vi "Response AutoControlRefHandler DataTypes.vi"() -> (3 "Unit Test Framework Results":T1)   [LabVIEW 2023]
uses:
  <vilib>/utf/common/utf_test_result_troll.ctl
  <vilib>/utf/common/utf_test_result.ctl
  <vilib>/utf/common/utf_test_result_failure.ctl
  <vilib>/utf/common/utf_test_comparison_operators.ctl
  <vilib>/utf/common/utf_vi_tag.ctl
  API Message/API Message.lvclass
  <vilib>/Utility/error.llb/DialogType.ctl
  <vilib>/httpClient/POSTBuffer.vi
  <vilib>/utf/NI_UnitTestFramework.lvlib
  Server/Server.lvclass
  <vilib>/httpClient/LabVIEWHTTPClient.lvlib
  <vilib>/Utility/Data Type/NI_Data Type.lvlib
panel:
  in  "Path Array":path[](array[path])=[path "C:/Program Files/National Instruments/CompactRIO", path "C:/Program Files/National Instruments/LabVIEW 2020", path "C:/Program Files/National Instruments/LabVIEW 2021", path "C:/Program Files/National Instruments/LabVIEW 2022", path "C:/Program Files/National Instruments/LabVIEW 2023", path "C:/Program Files/National Instruments/LabVIEW 2024", path "C:/Program Files/National Instruments/MAX", path "C:/Program Files/National Instruments/MXI", path "C:/Program Files/National Instruments/NI Controller Driver", path "C:/Program Files/National Instruments/NI Hardware Configuration", path "C:/Program Files/National Instruments/NI Package Manager", path "C:/Program Files/National Instruments/NI-DAQ", path "C:/Program Files/National Instruments/NI-PCNet", path "C:/Program Files/National Instruments/NI-QPXI", path "C:/Program Files/National Instruments/NI-Sync", path "C:/Program Files/National Instruments/NI-SyncBus", path "C:/Program Files/National Instruments/NI-SyncEnet", path "C:/Program Files/National Instruments/NI-TSU", path "C:/Program Files/National Instruments/PXI Platform Services", path "C:/Program Files/National Instruments/Real-Time Trace Viewer 2023", path "C:/Program Files/National Instruments/Shared"]
  in  "String Array":string[](array[string])=["C", "Program Files", "National Instruments"]
  in  "Boolean Array":bool[](array[boolean])=[FALSE, FALSE, FALSE, TRUE, FALSE, FALSE, TRUE, TRUE]
  in  "EXT Array":ext[](array[numeric])=[0.0, 3.456, 6.912, 10.368, 13.824, 17.279999999999999999, 20.736, 24.192, 27.648, 31.103999999999999999]
  in  "DBL Array":dbl[](array[numeric])=[0.0, 2.345, 4.69, 7.035, 9.38, 11.725000000000001, 14.07, 16.415000000000003, 18.76, 21.105]
  in  "SGL Array":sgl[](array[numeric])=[0.0, 1.234, 2.468, 3.702, 4.936, 6.17, 7.404, 8.638, 9.872, 11.106]
  in  "U64 Array":u64[](array[numeric])=[200000, 200001, 200002, 200003, 200004, 200005, 200006, 200007, 200008, 200009]
  in  "U32 Array":u32[](array[numeric])=[20000, 20001, 20002, 20003, 20004, 20005, 20006, 20007, 20008, 20009]
  in  "U16 Array":u16[](array[numeric])=[2000, 2001, 2002, 2003, 2004, 2005, 2006, 2007, 2008, 2009]
  in  "U8 Array":u8[](array[numeric])=[200, 201, 202, 203, 204, 205, 206, 207, 208, 209]
  in  "I64 Array":i64[](array[numeric])=[100000, 100001, 100002, 100003, 100004, 100005, 100006, 100007, 100008, 100009]
  in  "I32 Array":i32[](array[numeric])=[10000, 10001, 10002, 10003, 10004, 10005, 10006, 10007, 10008, 10009]
  in  "I16 Array":i16[](array[numeric])=[1000, 1001, 1002, 1003, 1004, 1005, 1006, 1007, 1008, 1009]
  in  "I8 Array":i8[](array[numeric])=[100, 101, 102, 103, 104, 105, 106, 107, 108, 109]
  in  "Path":path=path "C:/Program Files/National Instruments/LabVIEW 2020"
  in  "String":string="Hello, World!"
  in  "Boolean":bool
  in  "EXT":ext=11.0
  in  "DBL":dbl=10.0
  in  "SGL":sgl=9.0
  in  "U64":u8=8
  in  "I64":i8=4
  in  "U32":u8=7
  in  "I32":i8=3
  in  "U16":u8=6
  in  "I16":i8=2
  in  "U8":u8=5
  in  "I8":i8=1
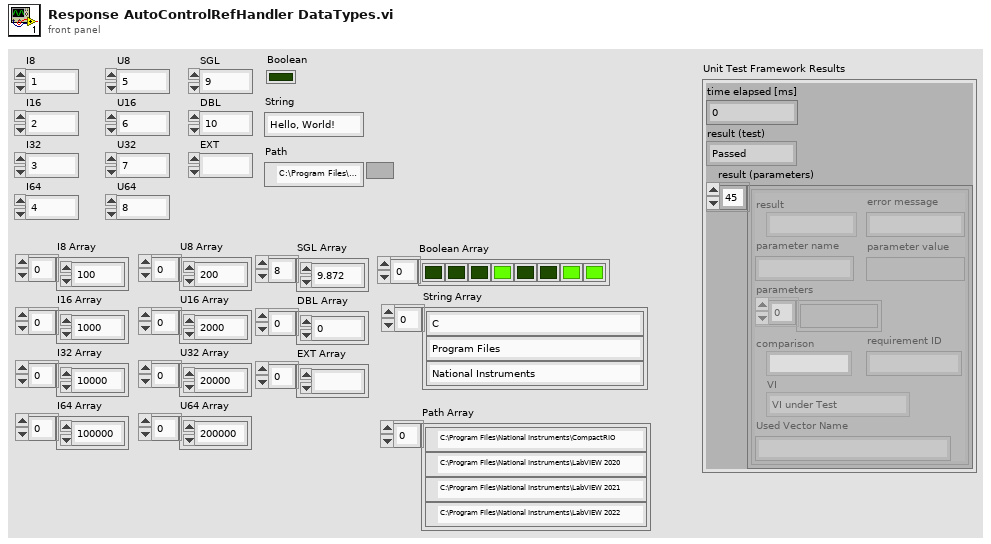
[diagram p1: front panel]
types:
  T1 = typedef "NI_UnitTestFramework.lvlib/utf_test_result_troll.ctl" = cluster{"time elapsed [ms]":u32, "result (test)":T2, "result (parameters)":T3[]}
  T2 = typedef "NI_UnitTestFramework.lvlib/utf_test_result.ctl" = enum16{"Passed", "Failed", "Error", "Skipped", "Not Processed"}
  T3 = typedef "NI_UnitTestFramework.lvlib/utf_test_result_failure.ctl" = cluster{"result":T2, "error message":string, "parameter name":string, "parameter value":variant, "parameters":variant[], "comparison":T4, "requirement ID":string, "VI":T5, "Used Vector Name":string}
  T4 = typedef "NI_UnitTestFramework.lvlib/utf_test_comparison_operators.ctl" = enum16{"=", "!=", ">", ">=", "<", "<=", "range", "symmetric tolerance", "asymmetric tolerance", "string contains", "string not contain", "array size", "string length", "array range", "by element", "array range (limit array)", "user-defined", "array contains", "array not contain", "vector length", "= (elm)", "!= (elm)", "= (case insensitive)", "!= (case insensitive)"}
  T5 = typedef "NI_UnitTestFramework.lvlib/utf_vi_tag.ctl" = enum16{"Setup VI", "VI under Test", "Teardown VI"}
  T6 = typedef "LabVIEWHTTPClient.lvlib/ClientHandle.ctl" = refnum<k1>
  T7 = typedef "DialogType.ctl" = u16
  T8 = typedef "NI_Data Type.lvlib/Data Type.ctl" = enum8{"Invalid Type", "Void", "I8", "I16", "I32", "I64", "U8", "U16", "U32", "U64", "Single Float", "Double Float", "Extended Float", "Single Complex", "Double Complex", "Extended Complex", "Enum U8", "Enum U16", "Enum U32", "Enum U64", "Single Float With Unit", "Double Float With Unit", "Extended Float With Unit", "Single Complex with Unit", "Double Complex with Unit", "Extended Complex with Unit", "Boolean", "String", "Path", "Picture", "Tag", "Array", "Cluster", "Variant", "LV Variant", "Waveform", "Timestamp", "Digital Waveform", "Digital Data", "ExpressData", "Refnum", "External Data", "VI", "Poly VI", "LabVIEW Class Instance", "Fixed Point", "Set Collection", "Map Collection"}
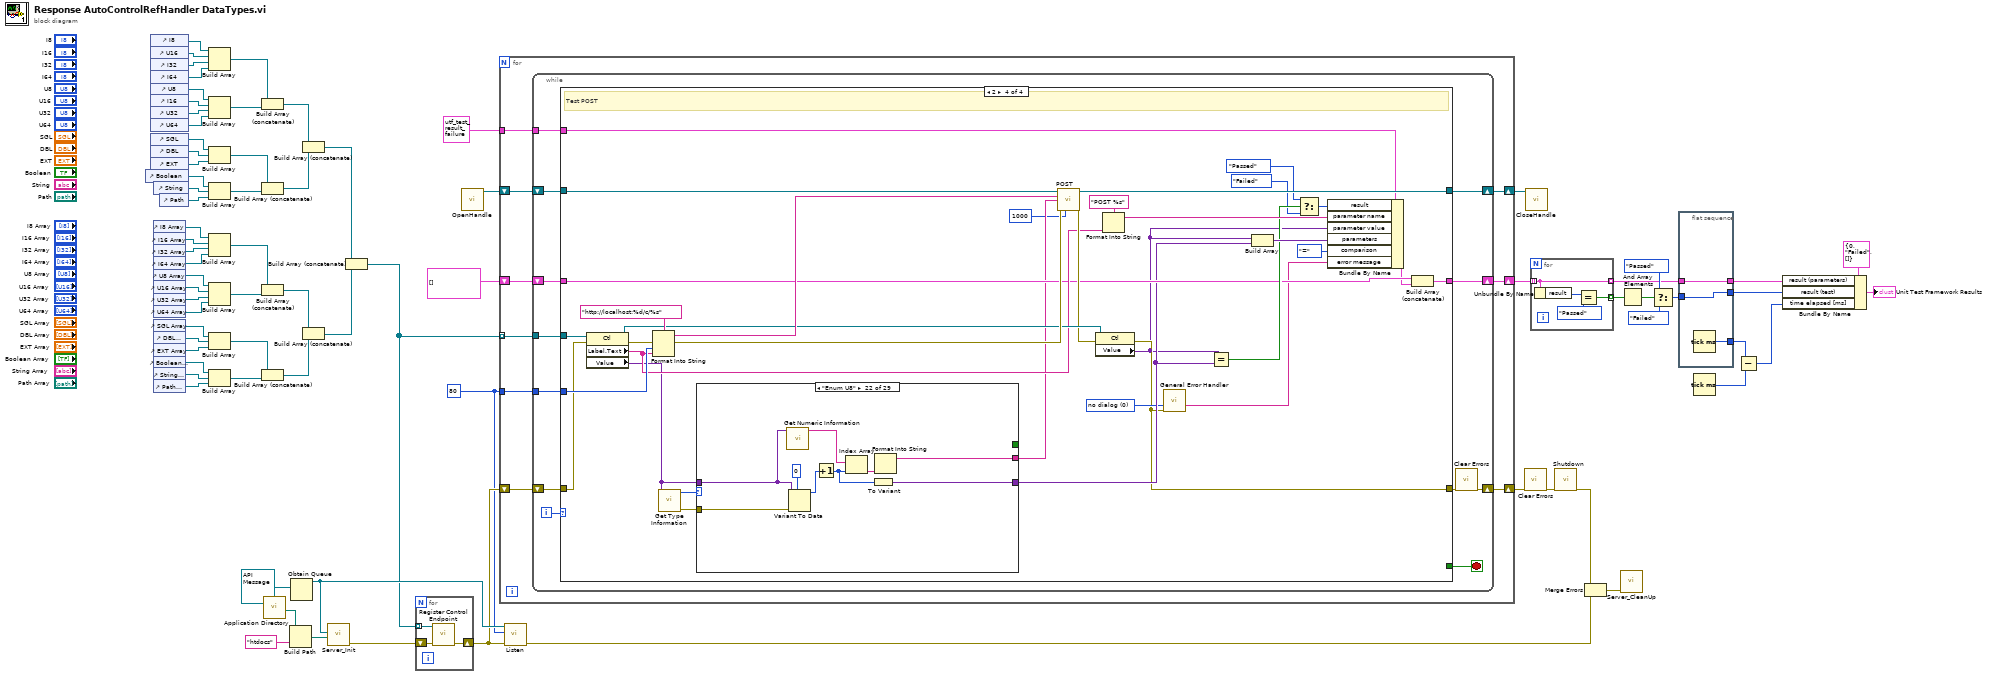
[diagram p0: block diagram]
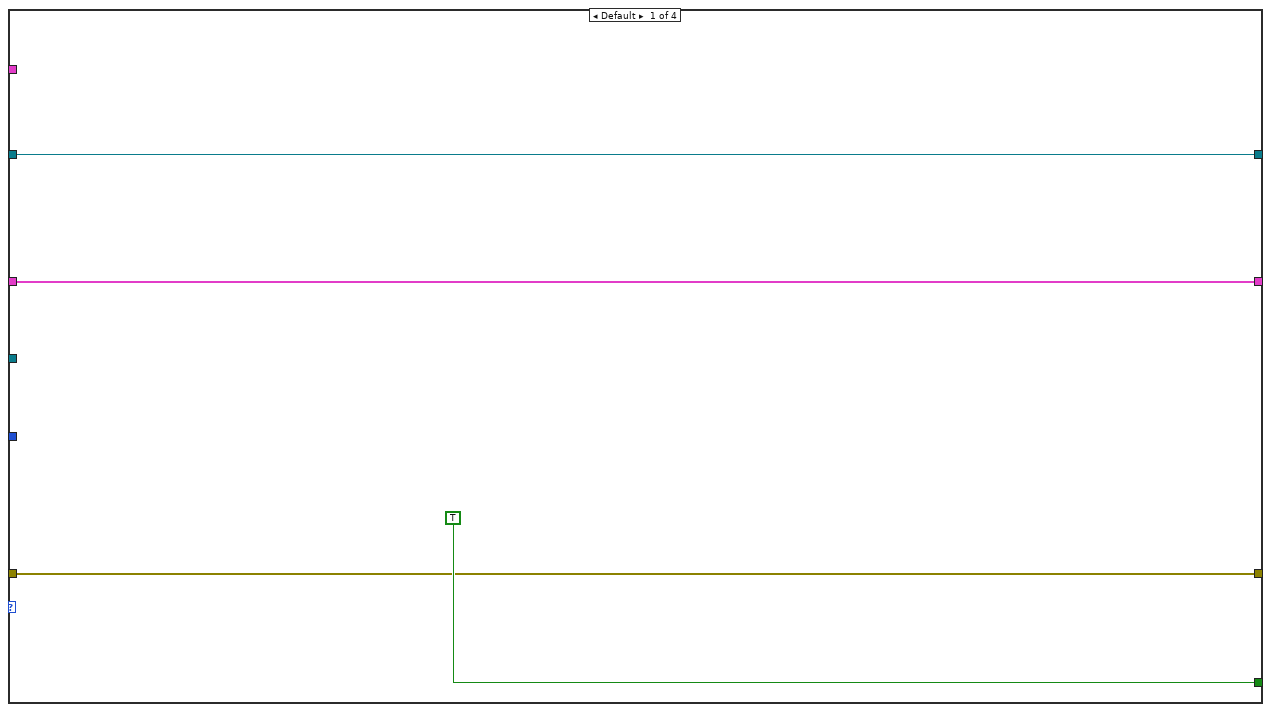
[diagram p2: hidden frame]
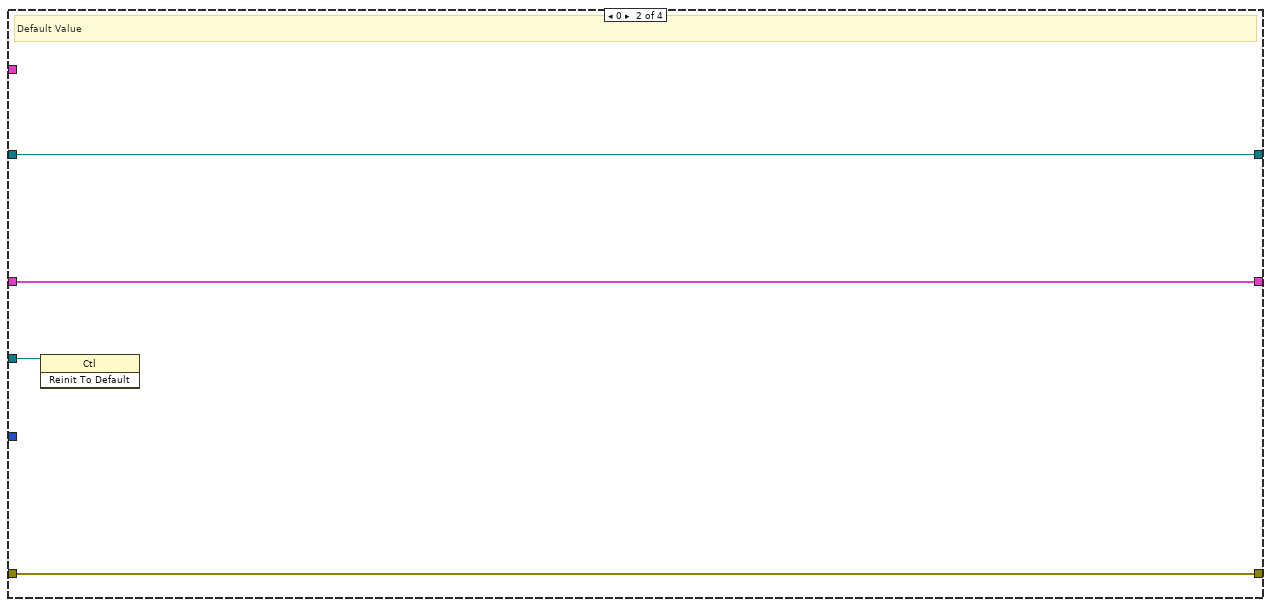
[diagram p3: hidden frame]
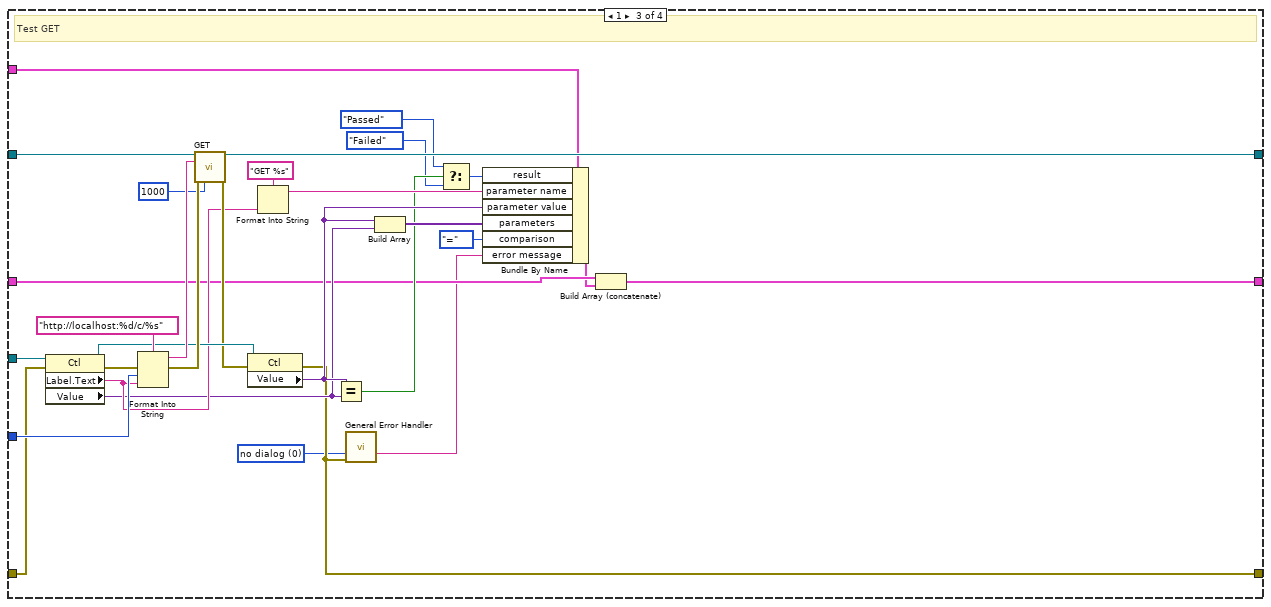
[diagram p4: hidden frame]
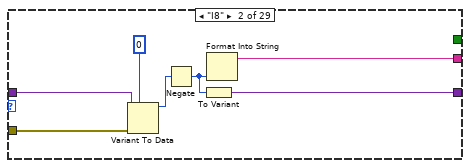
[diagram p6: hidden frame]
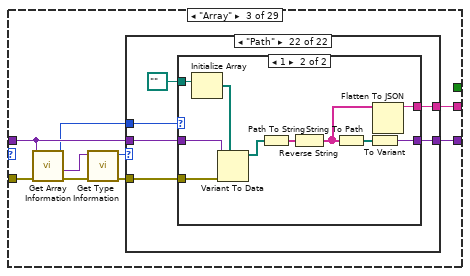
[diagram p7: hidden frame]
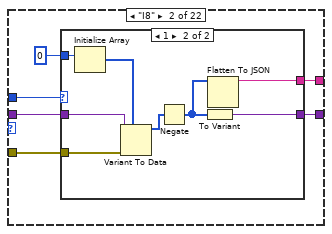
[diagram p9: hidden frame]
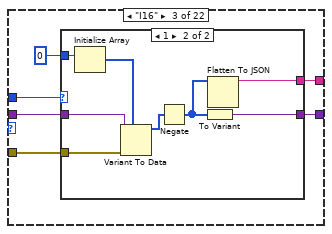
[diagram p11: hidden frame]
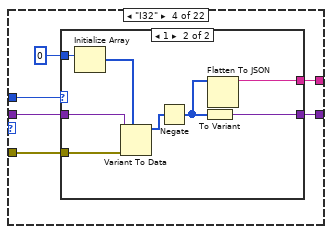
[diagram p13: hidden frame]
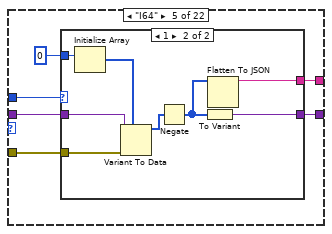
[diagram p15: hidden frame]
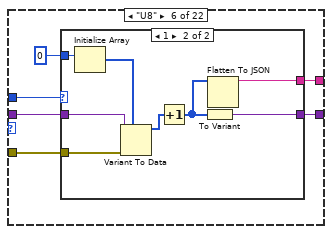
[diagram p17: hidden frame]
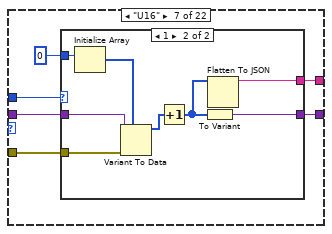
[diagram p19: hidden frame]
diagram:
  w33 = u16 80 ("Listen Port (80)")
  n1 = control-ref of="Boolean"() -> (w30:refnum<vi>)
  n2 = control-ref of="I8"() -> (w50:refnum<vi>)
  n3 = control-ref of="U16"() -> (w52:refnum<vi>)
  n4 = control-ref of="I32"() -> (w51:refnum<vi>)
  n5 = control-ref of="I64"() -> (w49:refnum<vi>)
  n6 = control-ref of="U8"() -> (w48:refnum<vi>)
  n7 = control-ref of="I16"() -> (w45:refnum<vi>)
  n8 = control-ref of="U32"() -> (w46:refnum<vi>)
  n9 = control-ref of="U64"() -> (w47:refnum<vi>)
  n10 = control-ref of="SGL"() -> (w35:refnum<vi>)
  n11 = control-ref of="DBL"() -> (w37:refnum<vi>)
  n12 = control-ref of="EXT"() -> (w36:refnum<vi>)
  n13 = control-ref of="String"() -> (w28:refnum<vi>)
  n14 = control-ref of="I8 Array"() -> (w8:refnum<vi>)
  n15 = control-ref of="I16 Array"() -> (w6:refnum<vi>)
  n16 = control-ref of="I32 Array"() -> (w7:refnum<vi>)
  n17 = control-ref of="I64 Array"() -> (w9:refnum<vi>)
  n18 = control-ref of="U8 Array"() -> (w10:refnum<vi>)
  n19 = control-ref of="U16 Array"() -> (w13:refnum<vi>)
  n20 = control-ref of="U32 Array"() -> (w12:refnum<vi>)
  n21 = control-ref of="U64 Array"() -> (w11:refnum<vi>)
  n22 = control-ref of="SGL Array"() -> (w16:refnum<vi>)
  n23 = control-ref of="DBL Array"() -> (w14:refnum<vi>)
  n24 = control-ref of="EXT Array"() -> (w15:refnum<vi>)
  n25 = control-ref of="Boolean Array"() -> (w17:refnum<vi>)
  n26 = control-ref of="String Array"() -> (w19:refnum<vi>)
  n27 = control-ref of="Path Array"() -> (w18:refnum<vi>)
  n28 = control-ref of="Path"() -> (w29:refnum<vi>)
  n29 = Build Array(w50, w52, w51, w49) -> (w67:refnum<vi>[])
  n30 = Build Array(w48, w45, w46, w47) -> (w66:refnum<vi>[])
  n31 = Build Array(w35, w37, w36) -> (w26:refnum<vi>[])
  n32 = Build Array(w30, w28, w29) -> (w27:refnum<vi>[])
  n33 = Build Array(w8, w6, w7, w9) -> (w4:refnum<vi>[])
  n34 = Build Array(w10, w13, w12, w11) -> (w5:refnum<vi>[])
  n35 = Build Array(w16, w14, w15) -> (w21:refnum<vi>[])
  n36 = Build Array(w17, w19, w18) -> (w20:refnum<vi>[])
  n37 = Build Array (concatenate)(w67, w66) -> (w24:refnum<vi>[])
  n38 = Build Array (concatenate)(w26, w27) -> (w25:refnum<vi>[])
  n39 = Build Array (concatenate)(w4, w5) -> (w23:refnum<vi>[])
  n40 = Build Array (concatenate)(w21, w20) -> (w22:refnum<vi>[])
  n41 = call <vilib>:"Application Directory.vi"() -> ("Application Directory"=w71:path)
  n42 = Build Path(base path=w71, name or relative path="htdocs" ("section")) -> (appended path=w70:path)
  n43 = Obtain Queue(element data type=refnum<class "API Message.lvclass"> refnum ("API Message.lvclass")) -> (queue out=w64:refnum<queue>)  [unwired: 4 in, 2 out]
  n44 = Build Array (concatenate)(w24, w25) -> (w2:refnum<vi>[])
  n45 = Build Array (concatenate)(w23, w22) -> (w3:refnum<vi>[])
  n46 = call "Server_Init.vi"("Static Data Folder"=w70, "API Queue"=w64) -> ("error out"=w68:errorcluster)  [unwired: 8 in, 1 out]
  n47 = Build Array (concatenate)(w2, w3) -> (w1:refnum<vi>[])
  n48 = for {
    shift-right: [w76] -> w63
    shift-left: w68 -> [w77]
    tunnel: w1 -> [w75] mode=indexing
    n49 = call "Register Control Endpoint.vi"("Error In"=w77, "Control Ref"=w75) -> ("Error Out"=w76:errorcluster)  [unwired: 9 in]
  }
  n50 = call <vilib>:"OpenHandle.vi"() -> ("client handle out"=w34:T6)  [unwired: 14 in, 1 out]
  n51 = for {
    tunnel: w1 -> [w82] mode=indexing
    shift-right: [w85] -> w57
    shift-left: T3[] [] ("result (parameters)") -> [w86]
    shift-right: [w83] -> w62
    shift-left: w63 -> [w84]
    shift-right: [w78] -> w31
    shift-left: w34 -> [w81]
    tunnel: w33 -> [w80]
    tunnel: T3 {"result"=enum."Not Processed", "error message"="", "parameter name"="", "parameter value"=variant, "parameters"=[], "comparison"=enum."=", "requirement ID"="", "VI"=enum."VI under Test", "Used Vector Name"=""} ("Unit Test Framework - result (parameters)") -> [w79]
    n52 = while {
      shift-right: [w96] -> w85
      shift-left: w86 -> [w97]
      shift-right: [w87] -> w83
      shift-left: w84 -> [w94]
      tunnel: w82 -> [w92]
      shift-right: [w90] -> w78
      shift-left: w81 -> [w91]
      tunnel: w80 -> [w89]
      tunnel: w79 -> [w88]
      i -> [w98]
      stop <- w95 stop-if-true
      n53 = case shown="2" w98 {
        tunnel: [TRUE _ _ _] -> w95
        tunnel: w97 -> [w101 w106 w112 w148]
        tunnel: [w101 w106 w113 w149] -> w96
        tunnel: w94 -> [w100 w105 w128 w162]
        tunnel: [w100 w105 w110 w140] -> w93
        tunnel: w92 -> [_ w104 w134 w168]
        tunnel: w91 -> [w99 w103 w135 w169]
        tunnel: [w99 w103 w136 w170] -> w90
        tunnel: w89 -> [_ _ w132 w166]
        tunnel: w88 -> [_ _ w121 w155]
        frame Default {
        }
        frame 0 {
          # "Default Value"
          n54 = invoke class="Ctl" method="Reinit To Default"(reference=w104) -> ()  [unwired: 2 in, 3 out]
        }
        frame 1 {
          w109 = T7 0 items=["no dialog", "OK message", "continue or stop message", "OK message + warnings", "continue/stop + warnings"] ("type of dialog (OK msg:1)")
          # "Test GET"
          n55 = property class="Ctl"(reference=w134, error in=w128) -> (reference out=w127:refnum<vi>, error out=w133:errorcluster, "Label.Text"=w125:string, "Value"=w119:variant)
          n56 = Format Into String(format string="http://localhost:%d/c/%s", error in=w133, w132, w125) -> (resulting string=w129:string, error out=w130:errorcluster)  [unwired: 1 in]
          n57 = call <vilib>:"GET.vi"("client handle"=w135, "url"=w129, "error in (no error)"=w130, "timeout (10000)"=1000) -> ("client handle out"=w136:T6, "error out"=w126:errorcluster)  [unwired: 8 in, 2 out]
          n58 = property class="Ctl"(reference=w127, error in=w126) -> (error out=w110:errorcluster, "Value"=w120:variant)  [unwired: 1 out]
          n59 = Format Into String(format string="GET %s", w125) -> (resulting string=w123:string)  [unwired: 2 in, 1 out]
          n60 = Equal?(x=w120, y=w119) -> (x = y?=w117:bool)
          n61 = call <vilib>:"General Error Handler.vi"("type of dialog (OK msg:1)"=w109, "error in (no error)"=w110) -> ("message"=w108:string)  [unwired: 9 in, 4 out]
          n62 = Build Array(w120, w119) -> (w118:variant[])
          n63 = Select(t=utf_test_result."Passed" ("y"), s=w117, f=utf_test_result."Failed" ("y")) -> (s? t:f=w114:T2)
          n64 = Bundle By Name(cluster=w121, "result"=w114, "parameter name"=w123, "parameter value"=w120, "parameters"=w118, "comparison"=utf_test_comparison_operators."=", "error message"=w108) -> (w111:T3)
          n65 = Build Array (concatenate)(w112, w111) -> (w113:T3[])
        }
        frame 2 {
          w141 = T7 0 items=["no dialog", "OK message", "continue or stop message", "OK message + warnings", "continue/stop + warnings"] ("type of dialog (OK msg:1)")
          # "Test POST"
          n66 = property class="Ctl"(reference=w168, error in=w162) -> (reference out=w161:refnum<vi>, error out=w167:errorcluster, "Label.Text"=w159:string, "Value"=w144:variant)
          n67 = Format Into String(format string="http://localhost:%d/c/%s", error in=w167, w166, w159) -> (resulting string=w163:string, error out=w164:errorcluster)  [unwired: 1 in]
          n68 = call <vilib>:"Get Type Information.vi"("variant"=w144) -> ("error out"=w145:errorcluster, "type"=w146:T8)  [unwired: 6 in, 3 out]
          n69 = case shown="\"Enum U8\"" w146 {
            tunnel: w145 -> [_ w178 w184 w548 w555 w564 w571 w578 w585 w593 w601 w609 w617 w625 w633 w641 w649 w657 w665 w673 w681 w690 w699 w708 w717 w724 w731 w738 w745]
            tunnel: w144 -> [w171 w172 w183 w542 w549 w558 w565 w572 w579 w587 w595 w603 w611 w619 w627 w635 w643 w651 w659 w667 w675 w685 w694 w703 w712 w718 w725 w732 w739]
            tunnel: [w171 w174 w187 w544 w551 w560 w567 w574 w581 w589 w597 w605 w613 w621 w629 w637 w645 w653 w661 w669 w677 w687 w696 w705 w714 w720 w727 w734 w741] -> w143
            tunnel: [_ w173 w186 w543 w550 w559 w566 w573 w580 w588 w596 w604 w612 w620 w628 w636 w644 w652 w660 w668 w676 w686 w695 w704 w713 w719 w726 w733 w740] -> w142
            tunnel: [_ _ _ _ _ _ _ _ _ TRUE TRUE TRUE TRUE TRUE TRUE TRUE TRUE TRUE TRUE TRUE TRUE _ _ _ _ _ _ _ _] -> _
            frame Default {
            }
            frame "I8" {
              n70 = Variant To Data(error in=w178, type=i8 0, Variant=w172) -> (data=w176:i8)  [unwired: 1 out]
              n71 = Negate(x=w176) -> (-x=w175:i8)
              n72 = To Variant(anything=w175) -> (Variant=w174:variant)
              n73 = Format Into String(w175) -> (resulting string=w173:string)  [unwired: 3 in, 1 out]
            }
            frame "Array" {
              n74 = call <vilib>:"Get Array Information.vi"("error in (no error)"=w184, "variant"=w183) -> ("error out"=w185:errorcluster, "array element data type"=w182:variant, "number of dimensions"=w181:i32)  [unwired: 6 in, 1 out]
              n75 = call <vilib>:"Get Type Information.vi"("error in (no error)"=w185, "variant"=w182) -> ("error out"=w180:errorcluster, "type"=w179:T8)  [unwired: 5 in, 3 out]
              n76 = case shown="\"Path\"" w179 {
                tunnel: [w188 w194 w209 w224 w239 w254 w269 w284 w299 w314 w329 w344 w359 w374 w389 w406 w429 w452 w475 w496 w515 w530] -> w187
                tunnel: [_ w193 w208 w223 w238 w253 w268 w283 w298 w313 w328 w343 w358 w373 w388 w405 w428 w451 w474 w495 w514 w529] -> w186
                tunnel: w183 -> [w188 w191 w206 w221 w236 w251 w266 w281 w296 w311 w326 w341 w356 w371 w386 w400 w423 w446 w469 w492 w511 w526]
                tunnel: w181 -> [_ w190 w205 w220 w235 w250 w265 w280 w295 w310 w325 w340 w355 w370 w385 w403 w426 w449 w472 w493 w512 w527]
                tunnel: w180 -> [_ w189 w204 w219 w234 w249 w264 w279 w294 w309 w324 w339 w354 w369 w384 w401 w424 w447 w470 w491 w510 w525]
                frame Default {
                }
                frame "I8" {
                  n77 = case shown="1" w190 {
                    tunnel: [w195 w202] -> w194
                    tunnel: [_ w201] -> w193
                    tunnel: w191 -> [w195 w200]
                    tunnel: i8 0 -> [_ w198]
                    tunnel: w189 -> [_ w199]
                    frame Default {
                    }
                    frame 1 {
                      n78 = Initialize Array(w198) -> (w197:i8[])  [unwired: 1 in]
                      n79 = Variant To Data(error in=w199, type=w197, Variant=w200) -> (data=w203:i8[])  [unwired: 1 out]
                      n80 = Negate(x=w203) -> (-x=w196:i8[])
                      n81 = To Variant(anything=w196) -> (Variant=w202:variant)
                      n82 = Flatten To JSON(anything=w196) -> (JSON string=w201:string)  [unwired: 2 in, 1 out]
                    }
                  }
                }
                frame "I16" {
                  n83 = case shown="1" w205 {
                    tunnel: [w210 w217] -> w209
                    tunnel: [_ w216] -> w208
                    tunnel: w206 -> [w210 w215]
                    tunnel: i16 0 -> [_ w213]
                    tunnel: w204 -> [_ w214]
                    frame Default {
                    }
                    frame 1 {
                      n84 = Initialize Array(w213) -> (w212:i16[])  [unwired: 1 in]
                      n85 = Variant To Data(error in=w214, type=w212, Variant=w215) -> (data=w218:i16[])  [unwired: 1 out]
                      n86 = Negate(x=w218) -> (-x=w211:i16[])
                      n87 = To Variant(anything=w211) -> (Variant=w217:variant)
                      n88 = Flatten To JSON(anything=w211) -> (JSON string=w216:string)  [unwired: 2 in, 1 out]
                    }
                  }
                }
                frame "I32" {
                  n89 = case shown="1" w220 {
                    tunnel: [w225 w232] -> w224
                    tunnel: [_ w231] -> w223
                    tunnel: w221 -> [w225 w230]
                    tunnel: 0 -> [_ w228]
                    tunnel: w219 -> [_ w229]
                    frame Default {
                    }
                    frame 1 {
                      n90 = Initialize Array(w228) -> (w227:i32[])  [unwired: 1 in]
                      n91 = Variant To Data(error in=w229, type=w227, Variant=w230) -> (data=w233:i32[])  [unwired: 1 out]
                      n92 = Negate(x=w233) -> (-x=w226:i32[])
                      n93 = To Variant(anything=w226) -> (Variant=w232:variant)
                      n94 = Flatten To JSON(anything=w226) -> (JSON string=w231:string)  [unwired: 2 in, 1 out]
                    }
                  }
                }
                frame "I64" {
                  n95 = case shown="1" w235 {
                    tunnel: [w240 w247] -> w239
                    tunnel: [_ w246] -> w238
                    tunnel: w236 -> [w240 w245]
                    tunnel: i64 0 -> [_ w243]
                    tunnel: w234 -> [_ w244]
                    frame Default {
                    }
                    frame 1 {
                      n96 = Initialize Array(w243) -> (w242:i64[])  [unwired: 1 in]
                      n97 = Variant To Data(error in=w244, type=w242, Variant=w245) -> (data=w248:i64[])  [unwired: 1 out]
                      n98 = Negate(x=w248) -> (-x=w241:i64[])
                      n99 = To Variant(anything=w241) -> (Variant=w247:variant)
                      n100 = Flatten To JSON(anything=w241) -> (JSON string=w246:string)  [unwired: 2 in, 1 out]
                    }
                  }
                }
                frame "U8" {
                  n101 = case shown="1" w250 {
                    tunnel: [w255 w262] -> w254
                    tunnel: [_ w261] -> w253
                    tunnel: w251 -> [w255 w260]
                    tunnel: u8 0 -> [_ w258]
                    tunnel: w249 -> [_ w259]
                    frame Default {
                    }
                    frame 1 {
                      n102 = Initialize Array(w258) -> (w257:u8[])  [unwired: 1 in]
                      n103 = Variant To Data(error in=w259, type=w257, Variant=w260) -> (data=w263:u8[])  [unwired: 1 out]
                      n104 = Increment(x=w263) -> (x+1=w256:u8[])
                      n105 = To Variant(anything=w256) -> (Variant=w262:variant)
                      n106 = Flatten To JSON(anything=w256) -> (JSON string=w261:string)  [unwired: 2 in, 1 out]
                    }
                  }
                }
                frame "U16" {
                  n107 = case shown="1" w265 {
                    tunnel: [w270 w277] -> w269
                    tunnel: [_ w276] -> w268
                    tunnel: w266 -> [w270 w275]
                    tunnel: u16 0 -> [_ w273]
                    tunnel: w264 -> [_ w274]
                    frame Default {
                    }
                    frame 1 {
                      n108 = Initialize Array(w273) -> (w272:u16[])  [unwired: 1 in]
                      n109 = Variant To Data(error in=w274, type=w272, Variant=w275) -> (data=w278:u16[])  [unwired: 1 out]
                      n110 = Increment(x=w278) -> (x+1=w271:u16[])
                      n111 = To Variant(anything=w271) -> (Variant=w277:variant)
                      n112 = Flatten To JSON(anything=w271) -> (JSON string=w276:string)  [unwired: 2 in, 1 out]
                    }
                  }
                }
                frame "U32" {
                  n113 = case shown="1" w280 {
                    tunnel: [w285 w292] -> w284
                    tunnel: [_ w291] -> w283
                    tunnel: w281 -> [w285 w290]
                    tunnel: u32 0 -> [_ w288]
                    tunnel: w279 -> [_ w289]
                    frame Default {
                    }
                    frame 1 {
                      n114 = Initialize Array(w288) -> (w287:u32[])  [unwired: 1 in]
                      n115 = Variant To Data(error in=w289, type=w287, Variant=w290) -> (data=w293:u32[])  [unwired: 1 out]
                      n116 = Increment(x=w293) -> (x+1=w286:u32[])
                      n117 = To Variant(anything=w286) -> (Variant=w292:variant)
                      n118 = Flatten To JSON(anything=w286) -> (JSON string=w291:string)  [unwired: 2 in, 1 out]
                    }
                  }
                }
                frame "U64" {
                  n119 = case shown="1" w295 {
                    tunnel: [w300 w307] -> w299
                    tunnel: [_ w306] -> w298
                    tunnel: w296 -> [w300 w305]
                    tunnel: u64 0 -> [_ w303]
                    tunnel: w294 -> [_ w304]
                    frame Default {
                    }
                    frame 1 {
                      n120 = Initialize Array(w303) -> (w302:u64[])  [unwired: 1 in]
                      n121 = Variant To Data(error in=w304, type=w302, Variant=w305) -> (data=w308:u64[])  [unwired: 1 out]
                      n122 = Increment(x=w308) -> (x+1=w301:u64[])
                      n123 = To Variant(anything=w301) -> (Variant=w307:variant)
                      n124 = Flatten To JSON(anything=w301) -> (JSON string=w306:string)  [unwired: 2 in, 1 out]
                    }
                  }
                }
                frame "Single Float" {
                  n125 = case shown="1" w310 {
                    tunnel: [w315 w322] -> w314
                    tunnel: [_ w321] -> w313
                    tunnel: w311 -> [w315 w320]
                    tunnel: sgl 0.0 -> [_ w318]
                    tunnel: w309 -> [_ w319]
                    frame Default {
                    }
                    frame 1 {
                      n126 = Initialize Array(w318) -> (w317:sgl[])  [unwired: 1 in]
                      n127 = Variant To Data(error in=w319, type=w317, Variant=w320) -> (data=w323:sgl[])  [unwired: 1 out]
                      n128 = Negate(x=w323) -> (-x=w316:sgl[])
                      n129 = To Variant(anything=w316) -> (Variant=w322:variant)
                      n130 = Flatten To JSON(anything=w316) -> (JSON string=w321:string)  [unwired: 2 in, 1 out]
                    }
                  }
                }
                frame "Single Float With Unit" {
                  n131 = case shown="1" w325 {
                    tunnel: [w330 w337] -> w329
                    tunnel: [_ w336] -> w328
                    tunnel: w326 -> [w330 w335]
                    tunnel: sgl 0.0 -> [_ w333]
                    tunnel: w324 -> [_ w334]
                    frame Default {
                    }
                    frame 1 {
                      n132 = Initialize Array(w333) -> (w332:sgl[])  [unwired: 1 in]
                      n133 = Variant To Data(error in=w334, type=w332, Variant=w335) -> (data=w338:sgl[])  [unwired: 1 out]
                      n134 = Negate(x=w338) -> (-x=w331:sgl[])
                      n135 = To Variant(anything=w331) -> (Variant=w337:variant)
                      n136 = Flatten To JSON(anything=w331) -> (JSON string=w336:string)  [unwired: 2 in, 1 out]
                    }
                  }
                }
                frame "Double Float" {
                  n137 = case shown="1" w340 {
                    tunnel: [w345 w352] -> w344
                    tunnel: [_ w351] -> w343
                    tunnel: w341 -> [w345 w350]
                    tunnel: 0.0 -> [_ w348]
                    tunnel: w339 -> [_ w349]
                    frame Default {
                    }
                    frame 1 {
                      n138 = Initialize Array(w348) -> (w347:dbl[])  [unwired: 1 in]
                      n139 = Variant To Data(error in=w349, type=w347, Variant=w350) -> (data=w353:dbl[])  [unwired: 1 out]
                      n140 = Negate(x=w353) -> (-x=w346:dbl[])
                      n141 = To Variant(anything=w346) -> (Variant=w352:variant)
                      n142 = Flatten To JSON(anything=w346) -> (JSON string=w351:string)  [unwired: 2 in, 1 out]
                    }
                  }
                }
                frame "Double Float With Unit" {
                  n143 = case shown="1" w355 {
                    tunnel: [w360 w367] -> w359
                    tunnel: [_ w366] -> w358
                    tunnel: w356 -> [w360 w365]
                    tunnel: 0.0 -> [_ w363]
                    tunnel: w354 -> [_ w364]
                    frame Default {
                    }
                    frame 1 {
                      n144 = Initialize Array(w363) -> (w362:dbl[])  [unwired: 1 in]
                      n145 = Variant To Data(error in=w364, type=w362, Variant=w365) -> (data=w368:dbl[])  [unwired: 1 out]
                      n146 = Negate(x=w368) -> (-x=w361:dbl[])
                      n147 = To Variant(anything=w361) -> (Variant=w367:variant)
                      n148 = Flatten To JSON(anything=w361) -> (JSON string=w366:string)  [unwired: 2 in, 1 out]
                    }
                  }
                }
                frame "Extended Float" {
                  n149 = case shown="1" w370 {
                    tunnel: [w375 w382] -> w374
                    tunnel: [_ w381] -> w373
                    tunnel: w371 -> [w375 w380]
                    tunnel: ext 0.0 -> [_ w378]
                    tunnel: w369 -> [_ w379]
                    frame Default {
                    }
                    frame 1 {
                      n150 = Initialize Array(w378) -> (w377:ext[])  [unwired: 1 in]
                      n151 = Variant To Data(error in=w379, type=w377, Variant=w380) -> (data=w383:ext[])  [unwired: 1 out]
                      n152 = Negate(x=w383) -> (-x=w376:ext[])
                      n153 = To Variant(anything=w376) -> (Variant=w382:variant)
                      n154 = Flatten To JSON(anything=w376) -> (JSON string=w381:string)  [unwired: 2 in, 1 out]
                    }
                  }
                }
                frame "Extended Float With Unit" {
                  n155 = case shown="1" w385 {
                    tunnel: [w390 w397] -> w389
                    tunnel: [_ w396] -> w388
                    tunnel: w386 -> [w390 w395]
                    tunnel: ext 0.0 -> [_ w393]
                    tunnel: w384 -> [_ w394]
                    frame Default {
                    }
                    frame 1 {
                      n156 = Initialize Array(w393) -> (w392:ext[])  [unwired: 1 in]
                      n157 = Variant To Data(error in=w394, type=w392, Variant=w395) -> (data=w398:ext[])  [unwired: 1 out]
                      n158 = Negate(x=w398) -> (-x=w391:ext[])
                      n159 = To Variant(anything=w391) -> (Variant=w397:variant)
                      n160 = Flatten To JSON(anything=w391) -> (JSON string=w396:string)  [unwired: 2 in, 1 out]
                    }
                  }
                }
                frame "Enum U8" {
                  n161 = call <vilib>:"Get Numeric Information.vi"("error in (no error)"=w401, "variant"=w400) -> ("error out"=w402:errorcluster, "enum names"=w399:string[])  [unwired: 6 in, 2 out]
                  n162 = case shown="1" w403 {
                    tunnel: [w407 w417] -> w406
                    tunnel: [_ w416] -> w405
                    tunnel: w400 -> [w407 w415]
                    tunnel: u8 0 -> [_ w413]
                    tunnel: w402 -> [_ w414]
                    tunnel: w399 -> [_ w411]
                    frame Default {
                    }
                    frame 1 {
                      n163 = Initialize Array(w413) -> (w412:u8[])  [unwired: 1 in]
                      n164 = Variant To Data(error in=w414, type=w412, Variant=w415) -> (data=w418:u8[])  [unwired: 1 out]
                      n165 = Increment(x=w418) -> (x+1=w410:u8[])
                      n166 = for {
                        tunnel: w411 -> [w421]
                        tunnel: w410 -> [w419] mode=indexing
                        tunnel: [w420] -> w409 mode=indexing
                        tunnel: [w419] -> w408 mode=indexing
                        n167 = Index Array(array=w421, index=w419) -> (element=w420:string)
                      }
                      n168 = To Variant(anything=w408) -> (Variant=w417:variant)
                      n169 = Flatten To JSON(anything=w409) -> (JSON string=w416:string)  [unwired: 2 in, 1 out]
                    }
                  }
                }
                frame "Enum U16" {
                  n170 = call <vilib>:"Get Numeric Information.vi"("error in (no error)"=w424, "variant"=w423) -> ("error out"=w425:errorcluster, "enum names"=w422:string[])  [unwired: 6 in, 2 out]
                  n171 = case shown="1" w426 {
                    tunnel: [w430 w440] -> w429
                    tunnel: [_ w439] -> w428
                    tunnel: w423 -> [w430 w438]
                    tunnel: u16 0 -> [_ w436]
                    tunnel: w425 -> [_ w437]
                    tunnel: w422 -> [_ w434]
                    frame Default {
                    }
                    frame 1 {
                      n172 = Initialize Array(w436) -> (w435:u16[])  [unwired: 1 in]
                      n173 = Variant To Data(error in=w437, type=w435, Variant=w438) -> (data=w441:u16[])  [unwired: 1 out]
                      n174 = Increment(x=w441) -> (x+1=w433:u16[])
                      n175 = for {
                        tunnel: w434 -> [w444]
                        tunnel: w433 -> [w442] mode=indexing
                        tunnel: [w443] -> w432 mode=indexing
                        tunnel: [w442] -> w431 mode=indexing
                        n176 = Index Array(array=w444, index=w442) -> (element=w443:string)
                      }
                      n177 = To Variant(anything=w431) -> (Variant=w440:variant)
                      n178 = Flatten To JSON(anything=w432) -> (JSON string=w439:string)  [unwired: 2 in, 1 out]
                    }
                  }
                }
                frame "Enum U32" {
                  n179 = call <vilib>:"Get Numeric Information.vi"("error in (no error)"=w447, "variant"=w446) -> ("error out"=w448:errorcluster, "enum names"=w445:string[])  [unwired: 6 in, 2 out]
                  n180 = case shown="1" w449 {
                    tunnel: [w453 w463] -> w452
                    tunnel: [_ w462] -> w451
                    tunnel: w446 -> [w453 w461]
                    tunnel: u32 0 -> [_ w459]
                    tunnel: w448 -> [_ w460]
                    tunnel: w445 -> [_ w457]
                    frame Default {
                    }
                    frame 1 {
                      n181 = Initialize Array(w459) -> (w458:u32[])  [unwired: 1 in]
                      n182 = Variant To Data(error in=w460, type=w458, Variant=w461) -> (data=w464:u32[])  [unwired: 1 out]
                      n183 = Increment(x=w464) -> (x+1=w456:u32[])
                      n184 = for {
                        tunnel: w457 -> [w467]
                        tunnel: w456 -> [w465] mode=indexing
                        tunnel: [w466] -> w455 mode=indexing
                        tunnel: [w465] -> w454 mode=indexing
                        n185 = Index Array(array=w467, index=w465) -> (element=w466:string)
                      }
                      n186 = To Variant(anything=w454) -> (Variant=w463:variant)
                      n187 = Flatten To JSON(anything=w455) -> (JSON string=w462:string)  [unwired: 2 in, 1 out]
                    }
                  }
                }
                frame "Enum U64" {
                  n188 = call <vilib>:"Get Numeric Information.vi"("error in (no error)"=w470, "variant"=w469) -> ("error out"=w471:errorcluster, "enum names"=w468:string[])  [unwired: 6 in, 2 out]
                  n189 = case shown="1" w472 {
                    tunnel: [w476 w486] -> w475
                    tunnel: [_ w485] -> w474
                    tunnel: w469 -> [w476 w484]
                    tunnel: u64 0 -> [_ w482]
                    tunnel: w471 -> [_ w483]
                    tunnel: w468 -> [_ w480]
                    frame Default {
                    }
                    frame 1 {
                      n190 = Initialize Array(w482) -> (w481:u64[])  [unwired: 1 in]
                      n191 = Variant To Data(error in=w483, type=w481, Variant=w484) -> (data=w487:u64[])  [unwired: 1 out]
                      n192 = Increment(x=w487) -> (x+1=w479:u64[])
                      n193 = for {
                        tunnel: w480 -> [w490]
                        tunnel: w479 -> [w488] mode=indexing
                        tunnel: [w489] -> w478 mode=indexing
                        tunnel: [w488] -> w477 mode=indexing
                        n194 = Index Array(array=w490, index=w488) -> (element=w489:string)
                      }
                      n195 = To Variant(anything=w477) -> (Variant=w486:variant)
                      n196 = Flatten To JSON(anything=w478) -> (JSON string=w485:string)  [unwired: 2 in, 1 out]
                    }
                  }
                }
                frame "Boolean" {
                  n197 = case shown="1" w493 {
                    tunnel: [w497 w506] -> w496
                    tunnel: [_ w505] -> w495
                    tunnel: w492 -> [w497 w504]
                    tunnel: FALSE -> [_ w502]
                    tunnel: w491 -> [_ w503]
                    frame Default {
                    }
                    frame 1 {
                      n198 = Initialize Array(w502) -> (w501:bool[])  [unwired: 1 in]
                      n199 = Variant To Data(error in=w503, type=w501, Variant=w504) -> (data=w507:bool[])  [unwired: 1 out]
                      n200 = Not(x=w507) -> (.not. x?=w500:bool[])
                      n201 = for {
                        tunnel: w500 -> [w509] mode=indexing
                        tunnel: [w509] -> w499 mode=indexing
                        tunnel: [w508] -> w498 mode=indexing
                        n202 = Format Into String(w509) -> (resulting string=w508:string)  [unwired: 3 in, 1 out]
                      }
                      n203 = To Variant(anything=w499) -> (Variant=w506:variant)
                      n204 = Flatten To JSON(anything=w498) -> (JSON string=w505:string)  [unwired: 2 in, 1 out]
                    }
                  }
                }
                frame "String" {
                  n205 = case shown="1" w512 {
                    tunnel: [w516 w523] -> w515
                    tunnel: [_ w522] -> w514
                    tunnel: w511 -> [w516 w521]
                    tunnel: "" -> [_ w519]
                    tunnel: w510 -> [_ w520]
                    frame Default {
                    }
                    frame 1 {
                      n206 = Initialize Array(w519) -> (w518:string[])  [unwired: 1 in]
                      n207 = Variant To Data(error in=w520, type=w518, Variant=w521) -> (data=w524:string[])  [unwired: 1 out]
                      n208 = Reverse String(1:w524) -> (0:w517:string[])
                      n209 = To Variant(anything=w517) -> (Variant=w523:variant)
                      n210 = Flatten To JSON(anything=w517) -> (JSON string=w522:string)  [unwired: 2 in, 1 out]
                    }
                  }
                }
                frame "Path" {
                  n211 = case shown="1" w527 {
                    tunnel: [w531 w540] -> w530
                    tunnel: [_ w539] -> w529
                    tunnel: w526 -> [w531 w538]
                    tunnel: path "" -> [_ w536]
                    tunnel: w525 -> [_ w537]
                    frame Default {
                    }
                    frame 1 {
                      n212 = Initialize Array(w536) -> (w535:path[])  [unwired: 1 in]
                      n213 = Variant To Data(error in=w537, type=w535, Variant=w538) -> (data=w541:path[])  [unwired: 1 out]
                      n214 = Path To String(path=w541) -> (string=w534:string[])
                      n215 = Reverse String(1:w534) -> (0:w532:string[])
                      n216 = String To Path(string=w532) -> (path=w533:path[])
                      n217 = To Variant(anything=w533) -> (Variant=w540:variant)
                      n218 = Flatten To JSON(anything=w532) -> (JSON string=w539:string)  [unwired: 2 in, 1 out]
                    }
                  }
                }
              }
            }
            frame "Boolean" {
              n219 = Variant To Data(error in=w548, type=FALSE, Variant=w542) -> (data=w546:bool)  [unwired: 1 out]
              n220 = Not(x=w546) -> (.not. x?=w545:bool)
              n221 = To Variant(anything=w545) -> (Variant=w544:variant)
              n222 = Format Into String(w545) -> (resulting string=w543:string)  [unwired: 3 in, 1 out]
            }
            frame "String" {
              n223 = Variant To Data(error in=w555, type="", Variant=w549) -> (data=w553:string)  [unwired: 1 out]
              n224 = Reverse String(1:w553) -> (0:w552:string)
              n225 = To Variant(anything=w552) -> (Variant=w551:variant)
              n226 = Format Into String(w552) -> (resulting string=w550:string)  [unwired: 3 in, 1 out]
            }
            frame "Path" {
              n227 = Variant To Data(error in=w564, type=path "", Variant=w558) -> (data=w562:path)  [unwired: 1 out]
              n228 = Path To String(path=w562) -> (string=w557:string)
              n229 = Reverse String(1:w557) -> (0:w561:string)
              n230 = String To Path(string=w561) -> (path=w556:path)
              n231 = To Variant(anything=w556) -> (Variant=w560:variant)
              n232 = Format Into String(w556) -> (resulting string=w559:string)  [unwired: 3 in, 1 out]
            }
            frame "I16" {
              n233 = Variant To Data(error in=w571, type=i16 0, Variant=w565) -> (data=w569:i16)  [unwired: 1 out]
              n234 = Negate(x=w569) -> (-x=w568:i16)
              n235 = To Variant(anything=w568) -> (Variant=w567:variant)
              n236 = Format Into String(w568) -> (resulting string=w566:string)  [unwired: 3 in, 1 out]
            }
            frame "I32" {
              n237 = Variant To Data(error in=w578, type=0, Variant=w572) -> (data=w576:i32)  [unwired: 1 out]
              n238 = Negate(x=w576) -> (-x=w575:i32)
              n239 = To Variant(anything=w575) -> (Variant=w574:variant)
              n240 = Format Into String(w575) -> (resulting string=w573:string)  [unwired: 3 in, 1 out]
            }
            frame "I64" {
              n241 = Variant To Data(error in=w585, type=i64 0, Variant=w579) -> (data=w583:i64)  [unwired: 1 out]
              n242 = Negate(x=w583) -> (-x=w582:i64)
              n243 = To Variant(anything=w582) -> (Variant=w581:variant)
              n244 = Format Into String(w582) -> (resulting string=w580:string)  [unwired: 3 in, 1 out]
            }
            frame "Single Float" {
              n245 = Variant To Data(error in=w593, type=sgl 0.0, Variant=w587) -> (data=w591:sgl)  [unwired: 1 out]
              n246 = Negate(x=w591) -> (-x=w590:sgl)
              n247 = To Variant(anything=w590) -> (Variant=w589:variant)
              n248 = Format Into String(w590) -> (resulting string=w588:string)  [unwired: 3 in, 1 out]
            }
            frame "Single Float With Unit" {
              n249 = Variant To Data(error in=w601, type=sgl 0.0, Variant=w595) -> (data=w599:sgl)  [unwired: 1 out]
              n250 = Negate(x=w599) -> (-x=w598:sgl)
              n251 = To Variant(anything=w598) -> (Variant=w597:variant)
              n252 = Format Into String(w598) -> (resulting string=w596:string)  [unwired: 3 in, 1 out]
            }
            frame "Double Float" {
              n253 = Variant To Data(error in=w609, type=0.0, Variant=w603) -> (data=w607:dbl)  [unwired: 1 out]
              n254 = Negate(x=w607) -> (-x=w606:dbl)
              n255 = To Variant(anything=w606) -> (Variant=w605:variant)
              n256 = Format Into String(w606) -> (resulting string=w604:string)  [unwired: 3 in, 1 out]
            }
            frame "Double Float With Unit" {
              n257 = Variant To Data(error in=w617, type=0.0, Variant=w611) -> (data=w615:dbl)  [unwired: 1 out]
              n258 = Negate(x=w615) -> (-x=w614:dbl)
              n259 = To Variant(anything=w614) -> (Variant=w613:variant)
              n260 = Format Into String(w614) -> (resulting string=w612:string)  [unwired: 3 in, 1 out]
            }
            frame "Extended Float" {
              n261 = Variant To Data(error in=w625, type=ext 0.0, Variant=w619) -> (data=w623:ext)  [unwired: 1 out]
              n262 = Negate(x=w623) -> (-x=w622:ext)
              n263 = To Variant(anything=w622) -> (Variant=w621:variant)
              n264 = Format Into String(w622) -> (resulting string=w620:string)  [unwired: 3 in, 1 out]
            }
            frame "Extended Float With Unit" {
              n265 = Variant To Data(error in=w633, type=ext 0.0, Variant=w627) -> (data=w631:ext)  [unwired: 1 out]
              n266 = Negate(x=w631) -> (-x=w630:ext)
              n267 = To Variant(anything=w630) -> (Variant=w629:variant)
              n268 = Format Into String(w630) -> (resulting string=w628:string)  [unwired: 3 in, 1 out]
            }
            frame "Single Complex" {
              n269 = Variant To Data(error in=w641, type=csg 0.0+0.0i, Variant=w635) -> (data=w639:csg)  [unwired: 1 out]
              n270 = Negate(x=w639) -> (-x=w638:csg)
              n271 = To Variant(anything=w638) -> (Variant=w637:variant)
              n272 = Format Into String(w638) -> (resulting string=w636:string)  [unwired: 3 in, 1 out]
            }
            frame "Single Complex with Unit" {
              n273 = Variant To Data(error in=w649, type=csg 0.0+0.0i, Variant=w643) -> (data=w647:csg)  [unwired: 1 out]
              n274 = Negate(x=w647) -> (-x=w646:csg)
              n275 = To Variant(anything=w646) -> (Variant=w645:variant)
              n276 = Format Into String(w646) -> (resulting string=w644:string)  [unwired: 3 in, 1 out]
            }
            frame "Double Complex" {
              n277 = Variant To Data(error in=w657, type=cdb 0.0+0.0i, Variant=w651) -> (data=w655:cdb)  [unwired: 1 out]
              n278 = Negate(x=w655) -> (-x=w654:cdb)
              n279 = To Variant(anything=w654) -> (Variant=w653:variant)
              n280 = Format Into String(w654) -> (resulting string=w652:string)  [unwired: 3 in, 1 out]
            }
            frame "Double Complex with Unit" {
              n281 = Variant To Data(error in=w665, type=cdb 0.0+0.0i, Variant=w659) -> (data=w663:cdb)  [unwired: 1 out]
              n282 = Negate(x=w663) -> (-x=w662:cdb)
              n283 = To Variant(anything=w662) -> (Variant=w661:variant)
              n284 = Format Into String(w662) -> (resulting string=w660:string)  [unwired: 3 in, 1 out]
            }
            frame "Extended Complex" {
              n285 = Variant To Data(error in=w673, type=cxt 0.0+0.0i, Variant=w667) -> (data=w671:cxt)  [unwired: 1 out]
              n286 = Negate(x=w671) -> (-x=w670:cxt)
              n287 = To Variant(anything=w670) -> (Variant=w669:variant)
              n288 = Format Into String(w670) -> (resulting string=w668:string)  [unwired: 3 in, 1 out]
            }
            frame "Extended Complex with Unit" {
              n289 = Variant To Data(error in=w681, type=cxt 0.0+0.0i, Variant=w675) -> (data=w679:cxt)  [unwired: 1 out]
              n290 = Negate(x=w679) -> (-x=w678:cxt)
              n291 = To Variant(anything=w678) -> (Variant=w677:variant)
              n292 = Format Into String(w678) -> (resulting string=w676:string)  [unwired: 3 in, 1 out]
            }
            frame "Enum U8" {
              n293 = call <vilib>:"Get Numeric Information.vi"("variant"=w685) -> ("enum names"=w684:string[])  [unwired: 7 in, 3 out]
              n294 = Variant To Data(error in=w690, type=u8 0, Variant=w685) -> (data=w688:u8)  [unwired: 1 out]
              n295 = Increment(x=w688) -> (x+1=w683:u8)
              n296 = Index Array(array=w684, index=w683) -> (element=w682:string)
              n297 = To Variant(anything=w683) -> (Variant=w687:variant)
              n298 = Format Into String(w682) -> (resulting string=w686:string)  [unwired: 3 in, 1 out]
            }
            frame "Enum U16" {
              n299 = call <vilib>:"Get Numeric Information.vi"("variant"=w694) -> ("enum names"=w693:string[])  [unwired: 7 in, 3 out]
              n300 = Variant To Data(error in=w699, type=u16 0, Variant=w694) -> (data=w697:u16)  [unwired: 1 out]
              n301 = Increment(x=w697) -> (x+1=w692:u16)
              n302 = Index Array(array=w693, index=w692) -> (element=w691:string)
              n303 = To Variant(anything=w692) -> (Variant=w696:variant)
              n304 = Format Into String(w691) -> (resulting string=w695:string)  [unwired: 3 in, 1 out]
            }
            frame "Enum U32" {
              n305 = call <vilib>:"Get Numeric Information.vi"("variant"=w703) -> ("enum names"=w702:string[])  [unwired: 7 in, 3 out]
              n306 = Variant To Data(error in=w708, type=u32 0, Variant=w703) -> (data=w706:u32)  [unwired: 1 out]
              n307 = Increment(x=w706) -> (x+1=w701:u32)
              n308 = Index Array(array=w702, index=w701) -> (element=w700:string)
              n309 = To Variant(anything=w701) -> (Variant=w705:variant)
              n310 = Format Into String(w700) -> (resulting string=w704:string)  [unwired: 3 in, 1 out]
            }
            frame "Enum U64" {
              n311 = call <vilib>:"Get Numeric Information.vi"("variant"=w712) -> ("enum names"=w711:string[])  [unwired: 7 in, 3 out]
              n312 = Variant To Data(error in=w717, type=u64 0, Variant=w712) -> (data=w715:u64)  [unwired: 1 out]
              n313 = Increment(x=w715) -> (x+1=w710:u64)
              n314 = Index Array(array=w711, index=w710) -> (element=w709:string)
              n315 = To Variant(anything=w710) -> (Variant=w714:variant)
              n316 = Format Into String(w709) -> (resulting string=w713:string)  [unwired: 3 in, 1 out]
            }
            frame "U8" {
              n317 = Variant To Data(error in=w724, type=u8 0, Variant=w718) -> (data=w722:u8)  [unwired: 1 out]
              n318 = Increment(x=w722) -> (x+1=w721:u8)
              n319 = To Variant(anything=w721) -> (Variant=w720:variant)
              n320 = Format Into String(w721) -> (resulting string=w719:string)  [unwired: 3 in, 1 out]
            }
            frame "U16" {
              n321 = Variant To Data(error in=w731, type=u16 0, Variant=w725) -> (data=w729:u16)  [unwired: 1 out]
              n322 = Increment(x=w729) -> (x+1=w728:u16)
              n323 = To Variant(anything=w728) -> (Variant=w727:variant)
              n324 = Format Into String(w728) -> (resulting string=w726:string)  [unwired: 3 in, 1 out]
            }
            frame "U32" {
              n325 = Variant To Data(error in=w738, type=u32 0, Variant=w732) -> (data=w736:u32)  [unwired: 1 out]
              n326 = Increment(x=w736) -> (x+1=w735:u32)
              n327 = To Variant(anything=w735) -> (Variant=w734:variant)
              n328 = Format Into String(w735) -> (resulting string=w733:string)  [unwired: 3 in, 1 out]
            }
            frame "U64" {
              n329 = Variant To Data(error in=w745, type=u64 0, Variant=w739) -> (data=w743:u64)  [unwired: 1 out]
              n330 = Increment(x=w743) -> (x+1=w742:u64)
              n331 = To Variant(anything=w742) -> (Variant=w741:variant)
              n332 = Format Into String(w742) -> (resulting string=w740:string)  [unwired: 3 in, 1 out]
            }
          }
          n333 = call-poly <vilib>:"POST.vi"("client handle"=w169, "url"=w163, "buffer"=w142, "error in (no error)"=w164, "timeout (10000)"=1000) -> ("client handle out"=w170:T6, "error out"=w160:errorcluster)  [unwired: 7 in, 2 out]
          n334 = property class="Ctl"(reference=w161, error in=w160) -> (error out=w140:errorcluster, "Value"=w137:variant)  [unwired: 1 out]
          n335 = Format Into String(format string="POST %s", w159) -> (resulting string=w157:string)  [unwired: 2 in, 1 out]
          n336 = call <vilib>:"General Error Handler.vi"("type of dialog (OK msg:1)"=w141, "error in (no error)"=w140) -> ("message"=w139:string)  [unwired: 9 in, 4 out]
          n337 = Equal?(x=w137, y=w143) -> (x = y?=w153:bool)
          n338 = Build Array(w137, w143) -> (w154:variant[])
          n339 = Select(t=utf_test_result."Passed" ("y"), s=w153, f=utf_test_result."Failed" ("y")) -> (s? t:f=w150:T2)
          n340 = Bundle By Name(cluster=w155, "result"=w150, "parameter name"=w157, "parameter value"=w137, "parameters"=w154, "comparison"=utf_test_comparison_operators."=", "error message"=w139) -> (w147:T3)
          n341 = Build Array (concatenate)(w148, w147) -> (w149:T3[])
        }
      }
      n342 = call <vilib>:"Clear Errors.vi"("error in (no error)"=w93) -> ("error out"=w87:errorcluster)  [unwired: 5 in, 1 out]
    }
  }
  n343 = call "Listen.vi"("error in (no error)"=w63, "Listen Port (80)"=w33, "API Queue"=w64) -> ("error out"=w59:errorcluster)  [unwired: 8 in]
  n344 = call <vilib>:"Clear Errors.vi"("error in (no error)"=w62) -> ("error out"=w61:errorcluster)  [unwired: 5 in, 1 out]
  n345 = call <vilib>:"CloseHandle.vi"("client handle"=w31) -> ()  [unwired: 14 in, 1 out]
  n346 = for {
    tunnel: w57 -> [w749] mode=indexing
    tunnel: [w749] -> w44 mode=indexing
    tunnel: [w746] -> w56 mode=indexing
    n347 = Unbundle By Name(w749) -> ("result"=w748:T2)
    n348 = Equal?(x=w748, y=utf_test_result."Passed") -> (x = y?=w746:bool)
  }
  n349 = call "Shutdown.vi"("error in (no error)"=w61) -> ("error out"=w60:errorcluster)  [unwired: 10 in]
  n350 = Merge Errors(w60, w59) -> (w58:errorcluster)
  n351 = call "Server_CleanUp.vi"("error in (no error)"=w58) -> ()  [unwired: 10 in, 1 out]
  n352 = And Array Elements(Boolean array=w56) -> (logical AND=w55:bool)
  n353 = Select(t=utf_test_result."Passed" ("y"), s=w55, f=utf_test_result."Failed" ("y")) -> (s? t:f=w43:T2)
  n354 = flat-sequence {
    tunnel: w44 -> [w751]
    tunnel: w43 -> [w752]
    tunnel: [w752] -> w42
    tunnel: [w751] -> w41
    tunnel: [w750] -> w40
    frame #0 {
      n355 = Tick Count (ms)() -> (millisecond timer value=w750:u32)
    }
  }
  n356 = Tick Count (ms)() -> (millisecond timer value=w39:u32)
  n357 = Subtract(x=w40, y=w39) -> (x-y=w38:u32)
  n358 = Bundle By Name(cluster=T1 {"time elapsed [ms]"=0, "result (test)"=enum."Failed", "result (parameters)"=[]} ("Unit Test Framework - Result"), "result (parameters)"=w41, "result (test)"=w42, "time elapsed [ms]"=w38) -> (→"Unit Test Framework Results":T1)
